vi "DAQ_GetRecord.vi"(8 "error in (no error)":errorcluster, 9 "Label":string, 10 "Task":string, 11 "Message Enqueuer":refnum<class "Message Enqueuer.lvclass">) -> (0 "error out":errorcluster, 3 "RecordData":T1 {"StopTime" format="%<%x %.3X>T"; "StartTime" format="%<%x %.3X>T"})   [LabVIEW 2025, in "DAQ_API.lvlib"]
uses:
  DAQ_API.lvlib
  <vilib>/ActorFramework/Message Enqueuer/Message Enqueuer.lvclass
  DAQ_Abstr/Task_Abstr/Task_Abstr/WaveformData.ctl
  DAQ_Module/DAQ_Module/DAQ_Module Messages/GetRecord Msg/GetRecord Msg.lvclass/GetRecord Msg.ctl
  <vilib>/ActorFramework/Message Enqueuer/Message Enqueuer.lvclass/Message Enqueuer.ctl
  <vilib>/ActorFramework/Message Enqueuer/Enqueue.vi
  DAQ_Module/DAQ_Module/DAQ_Module Messages/GetRecord Msg/GetRecord Msg.lvclass
  C:/Program Files (x86)/National Instruments/LabVIEW 2025/vi.lib/ActorFramework/Message/Message.lvclass
  <vilib>/ActorFramework/Message Priority Queue/Priority Enqueue.vi
  DAQ_Abstr/Task_Abstr/Task_Abstr/Task_Abstr.lvclass
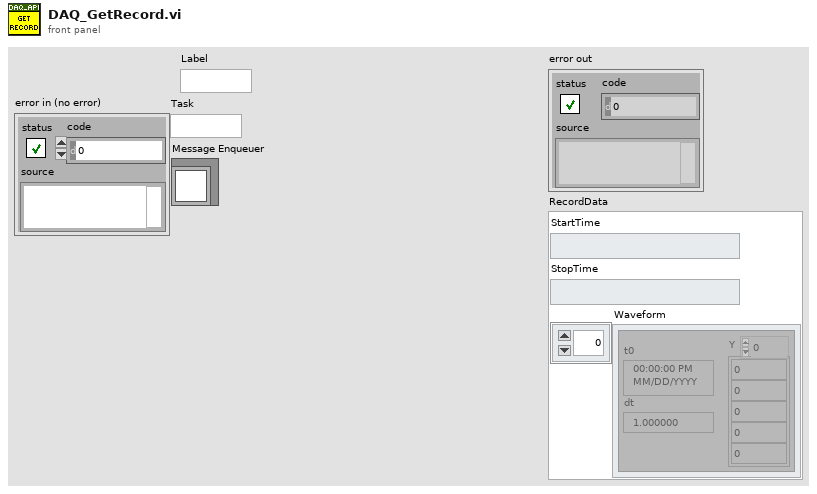
[diagram p1: front panel]
types:
  T1 = typedef "Task_Abstr.lvlib/Task_Abstr.lvclass/WaveformData.ctl" = cluster{"StartTime":timestamp, "StopTime":timestamp, "Waveform":waveform(dbl)[]}
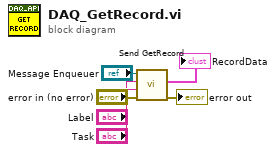
[diagram p0: block diagram]
diagram:
  n1 = call "Send GetRecord.vi"("error in (no error)"="error in (no error)", "Label"="Label", "Task"="Task", "Message Enqueuer"="Message Enqueuer") -> ("error out"=→"error out":errorcluster, "RecordData"=→"RecordData":T1)  [unwired: 5 in, 1 out]
